vi "Post-Build Action.vi"(5 "Files Generated by Build":path[](array[path]), 6 "Top Level/Always Included VIs":path[](array[path]), 7 "Destination Path":path, 8 "error in (no error)":errorcluster, 9 "Target Name":string, 10 "Build Specification Name":string, 11 "Project Path":path) -> (0 "error out":errorcluster)   [LabVIEW 2016]
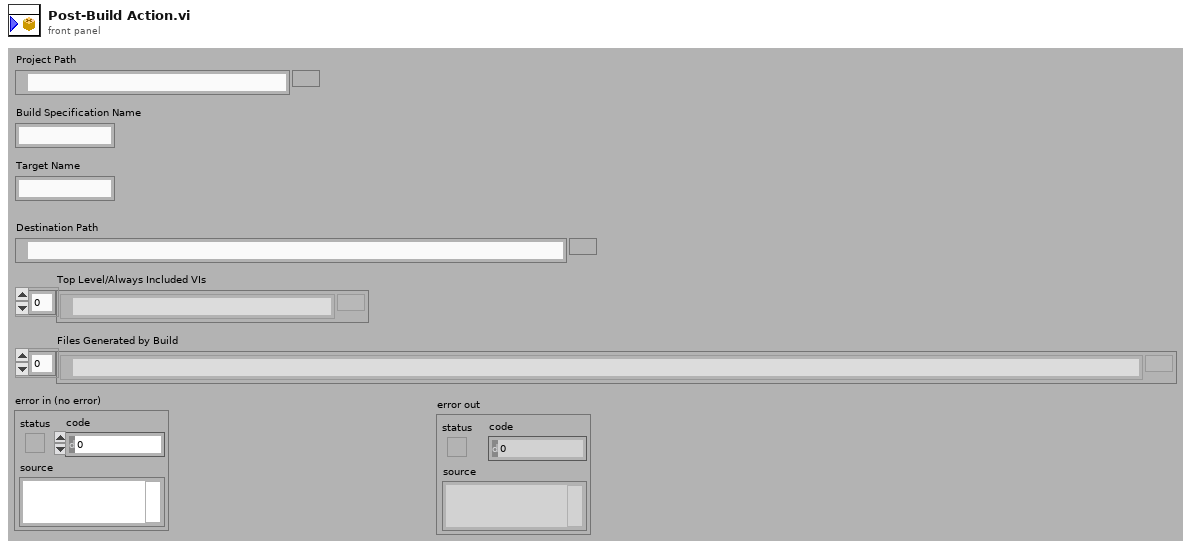
[diagram p1: front panel]
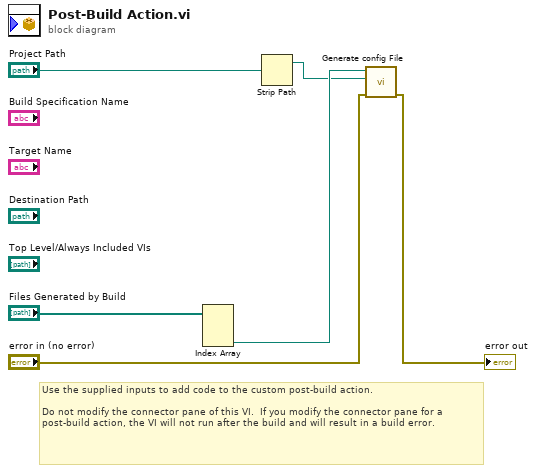
[diagram p0: block diagram]
diagram:
  # "Use the supplied inputs to add code to the custom post-build action.\n\nDo not modify the connector pane of this VI.  If you modify the connector pane for a post-build action, the VI will not run after the build and will result in a build error."
  n1 = Index Array(array="Files Generated by Build") -> (element #3=w2:path)  [unwired: 3 in, 2 out]
  n2 = Strip Path(path="Project Path") -> (stripped path=w1:path)  [unwired: 1 out]
  n3 = call "Generate config File.vi"("error in (no error)"="error in (no error)", "Path to top-level Directory"=w1, "Path to generated ini file"=w2) -> ("error out"=→"error out":errorcluster)  [unwired: 8 in]
